vi "GetRate.vi"(1 "Task ID":u32) -> (0 "return type":dbl)   [LabVIEW 2015]
uses:
  Windows/System32/AdvLvDaq.dll
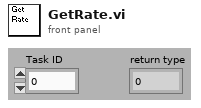
[diagram p1: front panel]
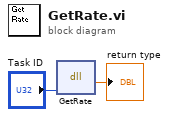
[diagram p0: block diagram]
diagram:
  n1 = dll-call lib="C:/Windows/System32/AdvLvDaq.dll" fn="GetRate"("taskId"="Task ID") -> ("return type"=→"return type":dbl)  [unwired: 4 in, 2 out]
